vi "Hardware Device Get All Info.vi"(8 "error in":errorcluster, 11 "NI Waveform Output in":refnum<class "NI Waveform Output.lvclass">) -> (0 "error out":errorcluster, 3 "NI Waveform Output out":refnum<class "NI Waveform Output.lvclass">)   [LabVIEW 2023, in "HardwareAbstractionLayer_LVOOP.lvlib" / "NI Waveform Output.lvclass"]
doc: "This VI Device Physical Channel Read"
uses:
  NI Waveform Output.lvclass
  NI Waveform Output.lvclass/NI Waveform Output.ctl
  <resource>/objmgr/daqmx.rc
panel:
  out "AO.WaveformPhysicalChans":tag[](array[tag])
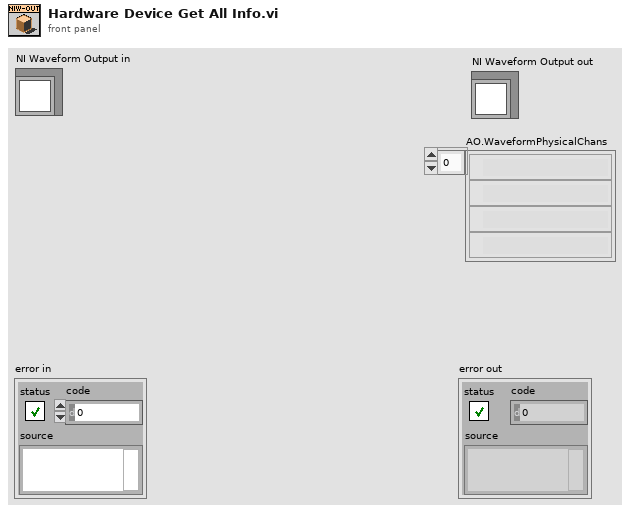
[diagram p1: front panel]
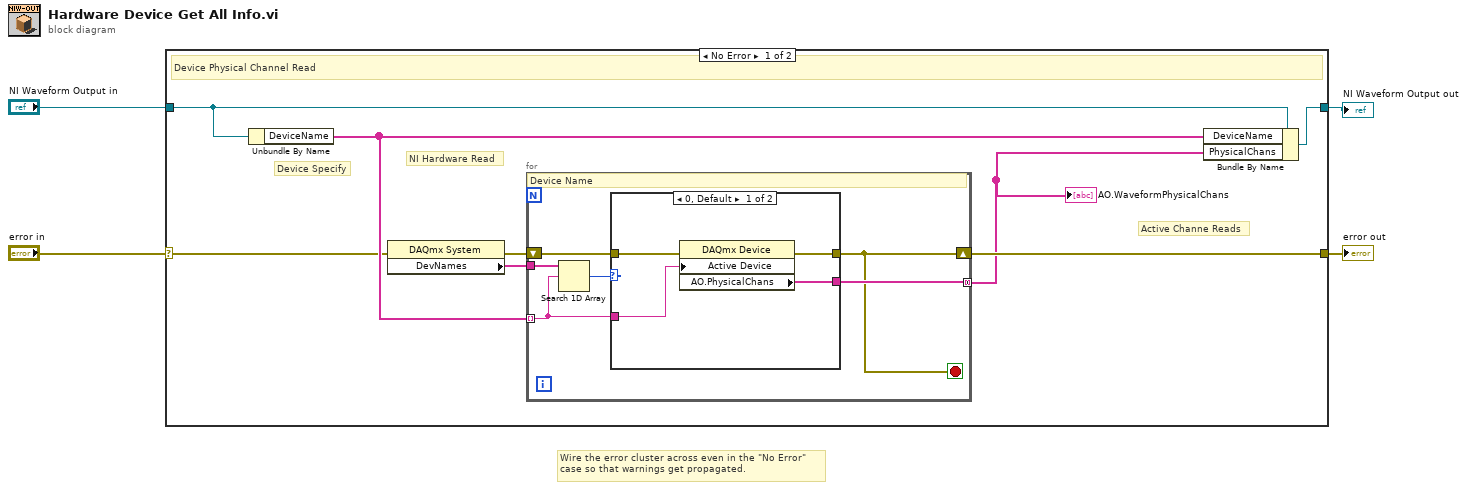
[diagram p0: block diagram]
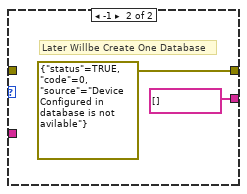
[diagram p2: hidden frame]
diagram:
  # "Wire the error cluster across even in the \"No Error\"\ncase so that warnings get propagated."
  n1 = case shown="No Error" "error in" {
    selector: "error in" -> [w6 w26]
    tunnel: [w8 w26] -> w3
    tunnel: [w7 w25] -> w1
    tunnel: "NI Waveform Output in" -> [w9 w25]
    frame No Error {
      # "Active Channe Reads"
      # "Device Specify"
      # "NI Hardware Read"
      # "Device Physical Channel Read"
      n2 = Unbundle By Name(w9) -> ("DeviceName"=w12:tag[])
      n3 = property class="DAQmx System"(error in=w6) -> (error out=w10:errorcluster, "DevNames"=w11:tag[])  [unwired: 1 in, 1 out]
      n4 = for {
        tunnel: w12 -> [w15] mode=indexing
        tunnel: w11 -> [w16]
        tunnel: [w14] -> w5 mode=concatenating
        shift-right: [w13] -> w8
        shift-left: w10 -> [w17]
        stop <- w13 stop-if-true
        # "Device Name"
        n5 = Search 1D Array(1D array=w16, element=w15) -> (index of element=w18:i32)  [unwired: 1 in]
        n6 = case shown="0, Default" w18 {
          tunnel: w17 -> [w20 _]
          tunnel: [w19 errorcluster {"status"=TRUE, "code"=0, "source"="Device  Configured in database is not avilable"} ("error out")] -> w13
          tunnel: w15 -> [w22 _]
          tunnel: [w21 tag[] [] ("AI.PhysicalChans")] -> w14
          frame 0, Default {
            n7 = property class="DAQmx Device"(error in=w20, "Active Device"=w22) -> (error out=w19:errorcluster, "AO.PhysicalChans"=w21:tag[])  [unwired: 1 in, 1 out]
          }
          frame -1 {
            # "Later Willbe Create One Database"
          }
        }
      }
      "AO.WaveformPhysicalChans" <- w5
      n8 = Bundle By Name(cluster=w9, "DeviceName"=w12, "PhysicalChans"=w5) -> (w7:refnum<class "NI Waveform Output.lvclass">)
    }
    frame Error {
    }
  }
  "error out" <- w3
  "NI Waveform Output out" <- w1
